vi "WriteParams.vi"(0 "CH1":dbl, 1 "CH5":dbl, 2 "CH6":dbl, 5 "CH2":dbl, 7 "CH3":dbl, 9 "CH4":dbl, 11 "error in (no error)":errorcluster, 12 "CH7":dbl, 13 "CH8":dbl) -> (15 "error out":errorcluster)   [LabVIEW 2014]
uses:
  <vilib>/addons/database/Connection.llb/DB Tools Open Connec (String).vi
  <vilib>/addons/database/Connection.llb/Conn Execute.vi
  <vilib>/addons/database/Recordset.llb/Rec Destroy - Connection.vi
  <vilib>/addons/database/NI_Database_API.lvlib
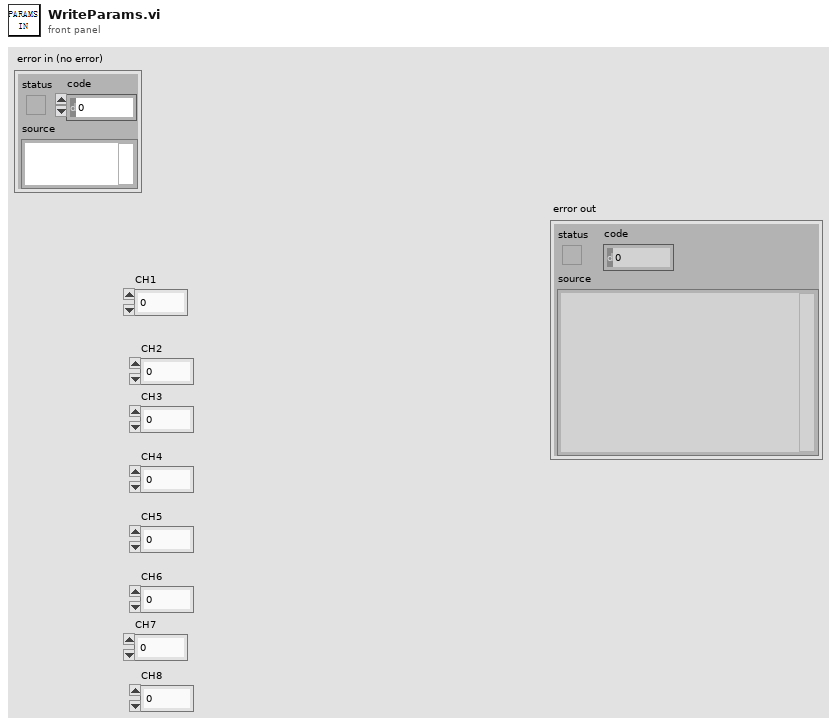
[diagram p1: front panel]
types:
  T1 = typedef "NI_Database_API.lvlib/Conn ObjectReference.ctl" = refnum<k1>
  T2 = typedef "NI_Database_API.lvlib/Rec ObjectReference.ctl" = refnum<k1>
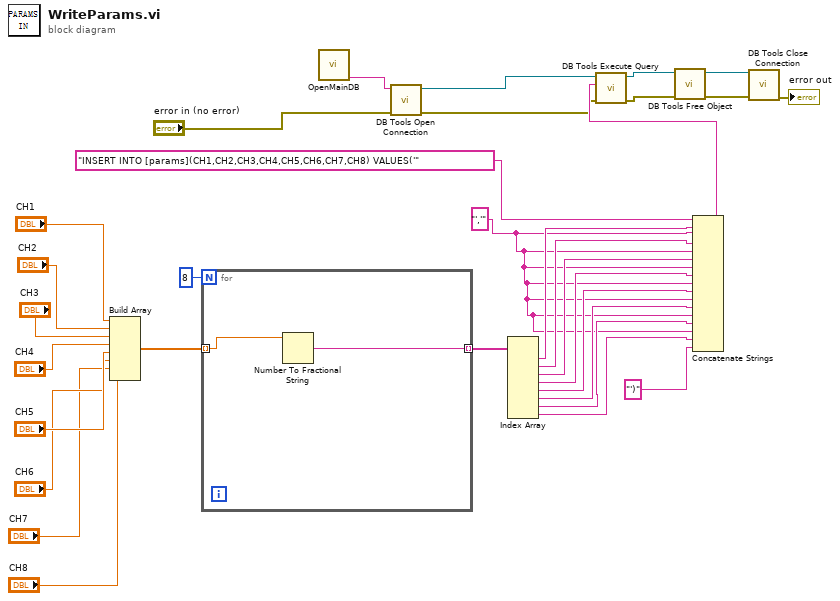
[diagram p0: block diagram]
diagram:
  w11 = "','"
  n1 = Build Array("CH1", "CH2", "CH3", "CH4", "CH5", "CH6", "CH7", "CH8") -> (w21:dbl[])
  n2 = for {
    N: 8 -> [_]
    tunnel: w21 -> [w34] mode=indexing
    tunnel: [w33] -> w20 mode=indexing
    n3 = Number To Fractional String(number=w34) -> (F-format string=w33:string)  [unwired: 3 in]
  }
  n4 = call "OpenMainDB.vi"() -> ("头信息"=w32:string)  [unwired: 11 in]
  n5 = call-poly <vilib>:"DB Tools Open Connection.vi"("error in (no error)"="error in (no error)", "connection information"=w32) -> ("error out"=w6:errorcluster, "connection reference"=w7:T1)  [unwired: 6 in]
  n6 = Index Array(array=w20) -> (element #1=w18:string, element #2=w17:string, element #3=w16:string, element #4=w15:string, element #5=w14:string, element #6=w13:string, element #7=w12:string, element #8=w10:string)  [unwired: 8 in]
  n7 = Concatenate Strings("INSERT INTO [params](CH1,CH2,CH3,CH4,CH5,CH6,CH7,CH8) VALUES('" ("SQL query"), w18, w11, w17, w11, w16, w11, w15, w11, w14, w11, w13, w11, w12, w11, w10, "')") -> (w8:string)
  n8 = call-poly <vilib>:"DB Tools Execute Query.vi"("error in (no error)"=w6, "SQL query"=w8, "connection reference"=w7) -> ("error out"=w4:errorcluster, "recordset reference"=w5:T2)  [unwired: 5 in]
  n9 = call-poly <vilib>:"DB Tools Free Object.vi"("error in (no error)"=w4, "recordset reference"=w5) -> ("error out"=w2:errorcluster, "connection reference"=w3:T1)  [unwired: 8 in]
  n10 = call <vilib>:"DB Tools Close Connection.vi"("error in (no error)"=w2, "connection reference"=w3) -> ("error out"=→"error out":errorcluster)  [unwired: 5 in]
